vi "JJMCclase12p2.vi"() -> ()   [LabVIEW 2013]
panel:
  out "Suma de arreglos":dbl
  out "numeros":dbl[](array[numeric])
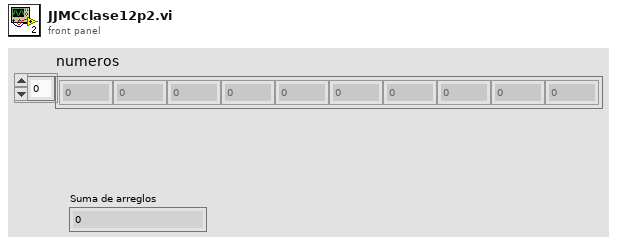
[diagram p1: front panel]
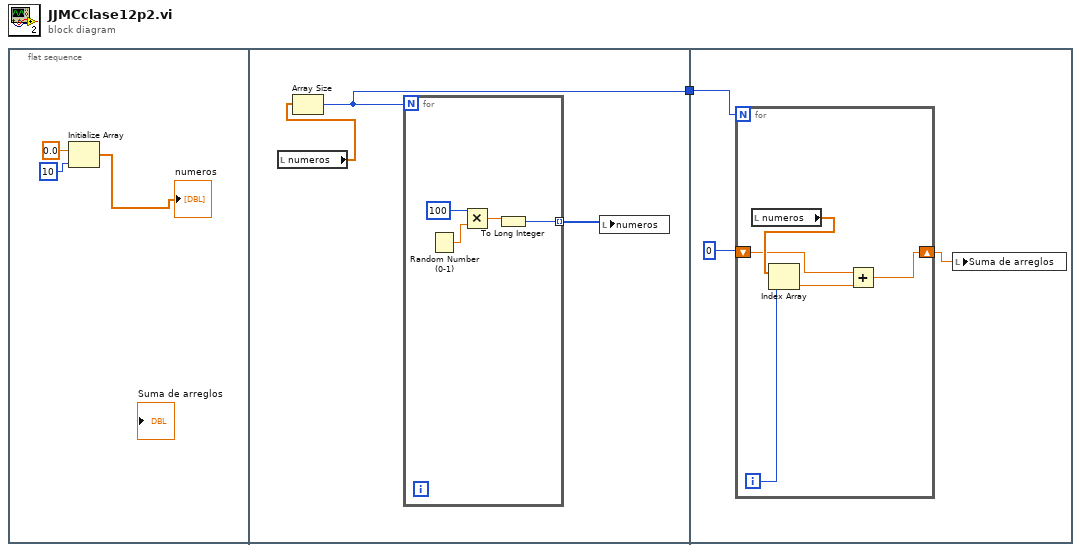
[diagram p0: block diagram]
diagram:
  n1 = flat-sequence {
    tunnel: [w5] -> w1
    tunnel: w1 -> [w14]
    frame #0 {
      n2 = Initialize Array(0.0 ("element"), 10) -> (→"numeros":dbl[])
    }
    frame #1 {
      n3 = local read "numeros"() -> (w7:dbl[])
      n4 = Array Size(array=w7) -> (size(s)=w5:i32)
      n5 = for {
        N: w5 -> [_]
        tunnel: [w8] -> w6 mode=indexing
        n6 = Random Number (0-1)() -> (number: 0 to 1=w10:dbl)
        n7 = Multiply(x=100, y=w10) -> (x*y=w9:dbl)
        n8 = To Long Integer(number=w9) -> (32bit integer=w8:i32)
      }
      n9 = local write "numeros"(w6) -> ()
    }
    frame #2 {
      n10 = for {
        N: w14 -> [_]
        shift-right: [w15] -> w12
        shift-left: 0 -> [w16]
        i -> [w19]
        n11 = local read "numeros"() -> (w18:dbl[])
        n12 = Index Array(array=w18, index=w19) -> (element=w17:dbl)
        n13 = Add(x=w16, y=w17) -> (x+y=w15:dbl)
      }
      n14 = local write "Suma de arreglos"(w12) -> ()
    }
  }
